vi "LabVIEWArduino1SpreadSheet.vi"() -> ()   [LabVIEW 2020]
uses:
  <vilib>/Instr/_visa.llb/VISA Configure Serial Port (Instr).vi
panel:
  out "FOUND STRING":i32
  out "Element 2":dbl[](array[numeric]) caption="Temperature Array"
  out "Second Element 2":dbl[](graph)
  in  "write buffer":string
  out "GO DOWN ECHO 2":string
  out "GO UP ECHO":string
  in  "GO UP":bool
  in  "GO DOWN":bool
  out "MAX SPEED ECHO":string
  out "SLOW SPEED ECHO":string
  in  "MAX SPEED":bool
  in  "SLOWEST SPEED":bool
  out "First Element":dbl[](graph)
  in  "VISA resource name":refnum<visa-resource-name>="COM3"
  in  "data bits (8)":u16=8 min=5 max=8 step=1
  in  "stop bits (10: 1 bit)":u16(ring)=10 items=["1.0"=10, "1.5"=15, "2.0"=20]
  in  "flow control (0:none)":u16(ring) items=["None", "XON/XOFF", "RTS/CTS", "XON/XOFF & RTS/CTS", "DTR/DSR", "XON/XOFF & DTR/DSR"]
  in  "parity (0:none)":enum16{"None", "Odd", "Even", "Mark", "Space"}(ring)
  out "Element 1":dbl[](array[numeric]) caption="Temperature Array"
  out "concatenated string":string
  in  "stop":bool
  in  "LabVIEW Stop":bool
  out "LabVIEW Echo":string
  out "Emergency Stop Echo":string
  in  "Emergency Stop!":bool
  out "DECELLERATE ECHO":string
  in  "Decellerate":bool
  in  "Motor Control Duino":refnum<visa-resource-name>
  in  "Accelerate":bool
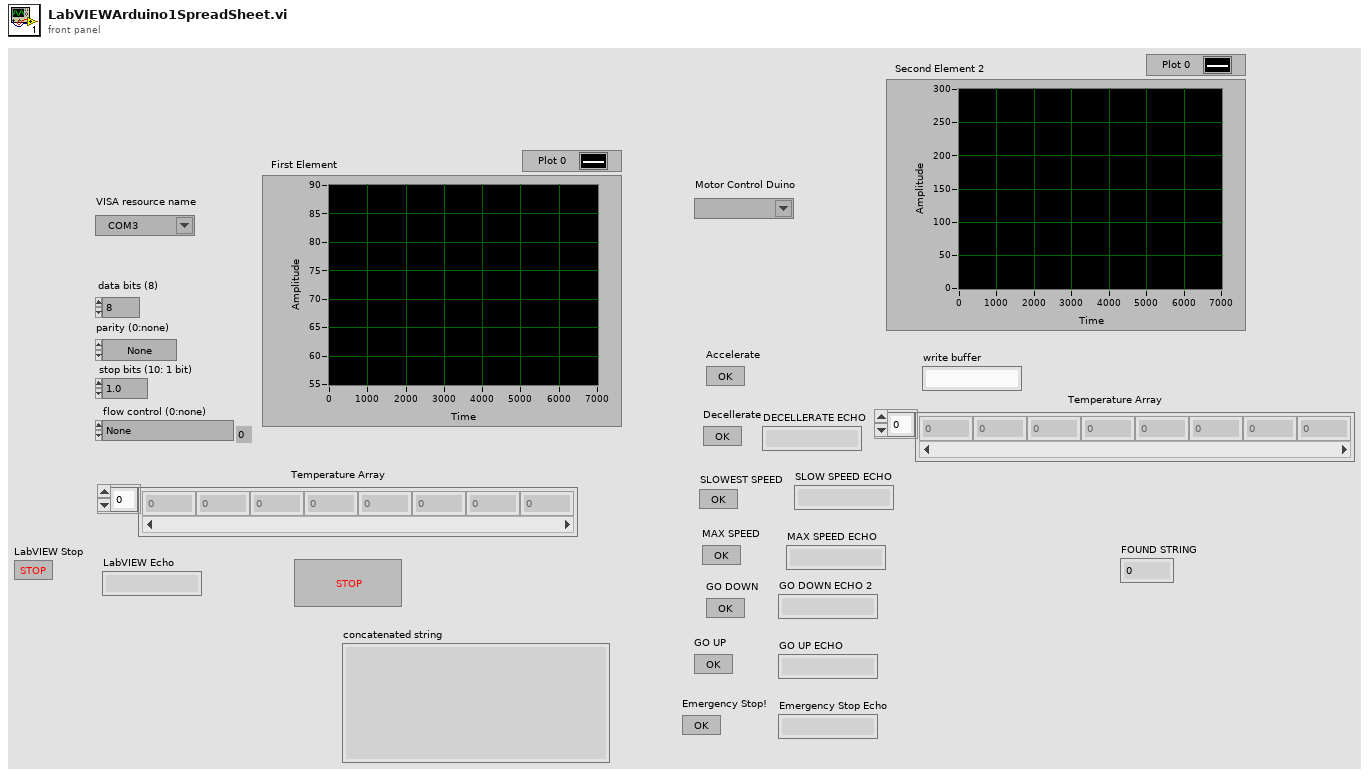
[diagram p1: front panel]
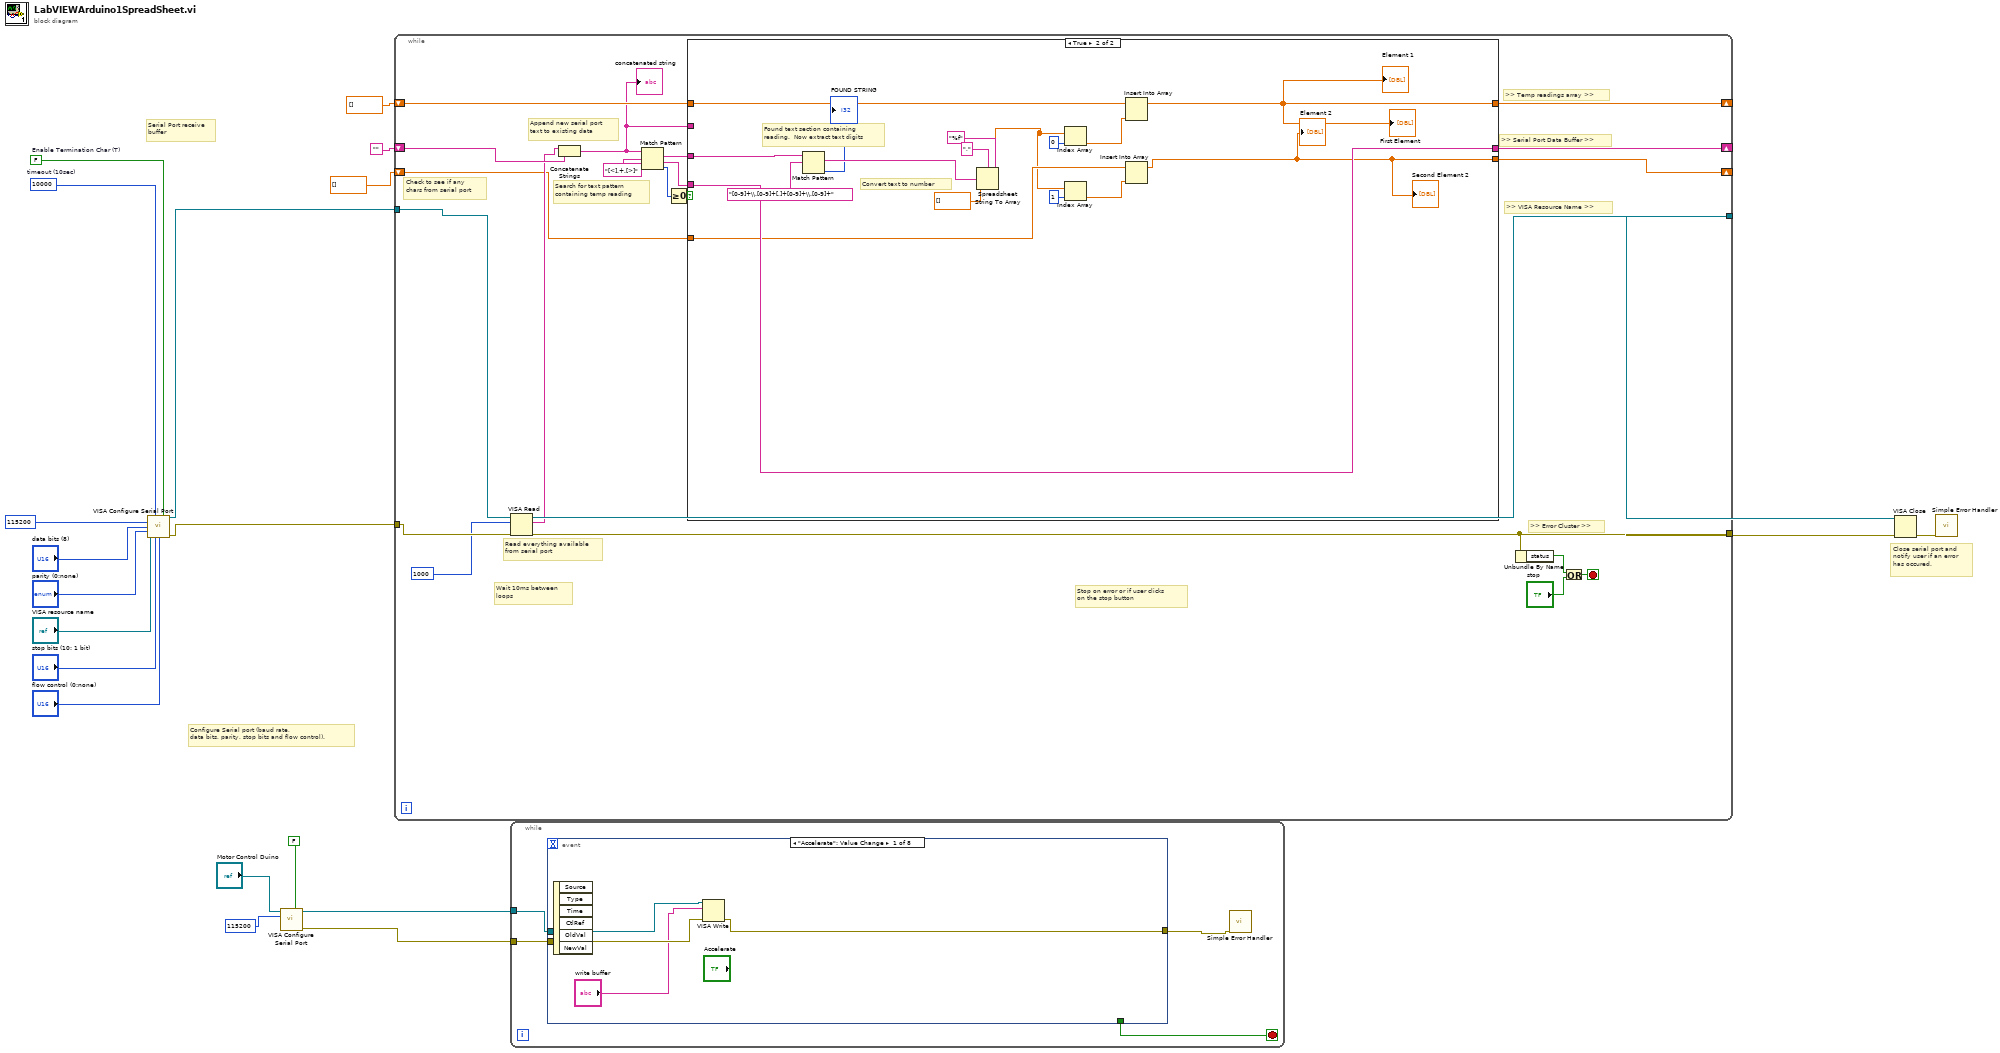
[diagram p0: block diagram]
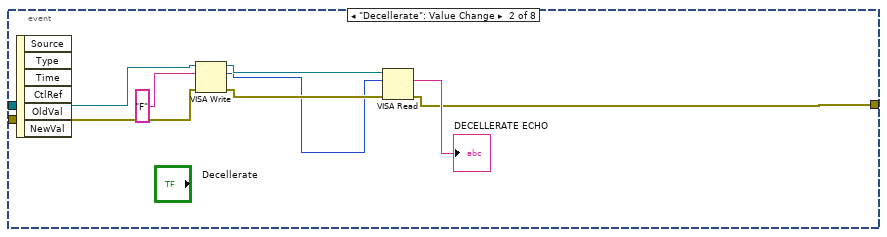
[diagram p3: hidden frame]
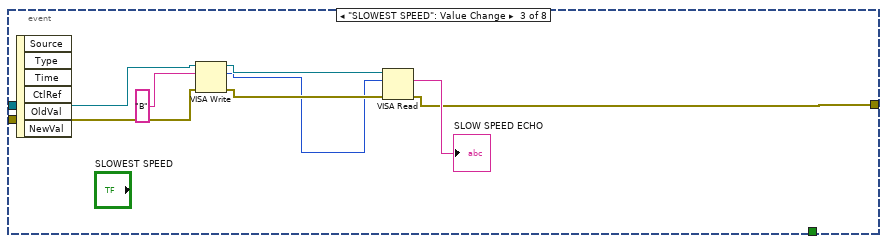
[diagram p4: hidden frame]
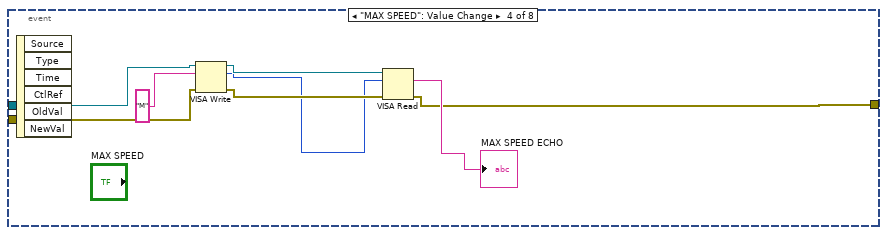
[diagram p5: hidden frame]
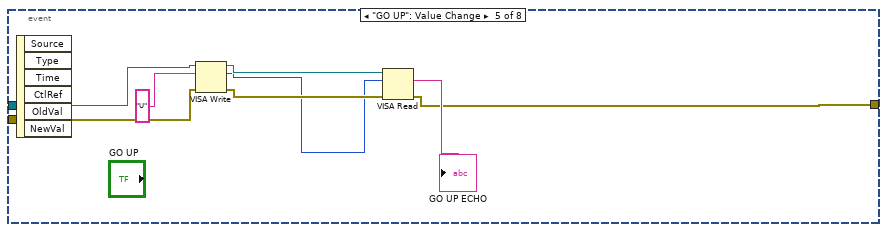
[diagram p6: hidden frame]
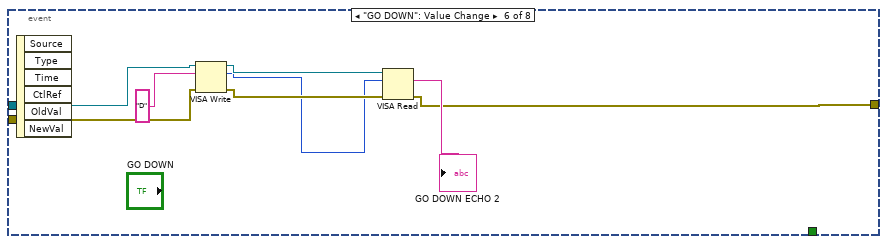
[diagram p7: hidden frame]
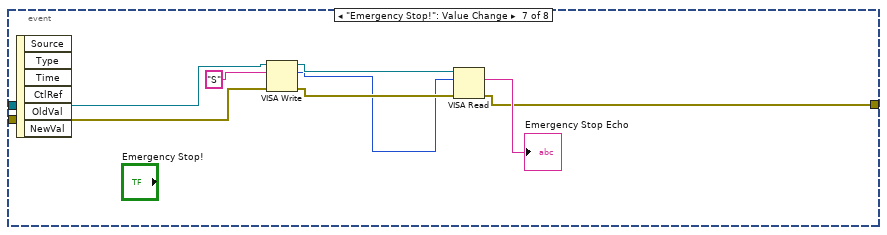
[diagram p8: hidden frame]
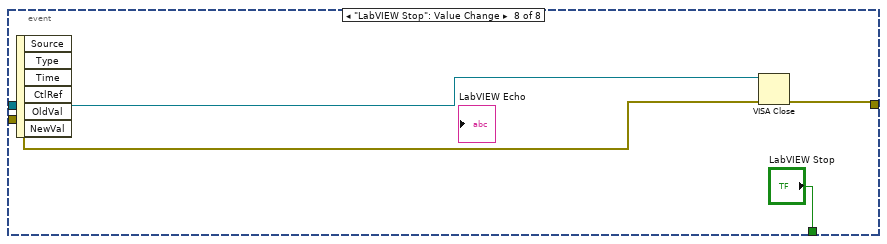
[diagram p9: hidden frame]
diagram:
  w13 = FALSE  # Enable Termination Char (T)
  w14 = u32 10000  # timeout (10sec)
  # "Close serial port and\nnotify user if an error\nhas occured."
  # "Serial Port receive\nbuffer"
  # "Configure Serial port (baud rate,\ndata bits, parity, stop bits and flow control)."
  n1 = call-poly "VISA Configure Serial Port"("VISA resource name"="VISA resource name", "timeout (10sec)"=w14, "Enable Termination\nChar (T)"=w13, "baud rate (9600)"=u32 115200, "data bits (8)"="data bits (8)", "parity (0:none)"="parity (0:none)", "stop bits (10: 1 bit)"="stop bits (10: 1 bit)", "flow control (0:none)"="flow control (0:none)") -> ("VISA resource name out"=w4:refnum<visa-resource-name>, "error out"=w3:errorcluster)  [unwired: 6 in]
  n2 = call-poly "VISA Configure Serial Port"("VISA resource name"="Motor Control Duino", "Enable Termination\nChar (T)"=FALSE ("Enable Termination\nChar (T)"), "baud rate (9600)"=u32 115200) -> ("VISA resource name out"=w21:refnum<visa-resource-name>, "error out"=w20:errorcluster)  [unwired: 11 in]
  n3 = while {
    tunnel: [w40] -> w17
    tunnel: [w42] -> w16
    shift-right: [w34] -> _
    shift-left: "" -> [w41]
    shift-right: [w36] -> _
    shift-left: dbl[] [] -> [w35]
    tunnel: w4 -> [w33]
    tunnel: w3 -> [w32]
    shift-right: [w23] -> _
    shift-left: dbl[] [] -> [w22]
    stop <- w39 stop-if-true
    # "Search for text pattern\ncontaining temp reading"
    # "Append new serial port\ntext to existing data"
    # "Read everything available\nfrom serial port"
    # "Wait 10ms between \nloops"
    # "Stop on error or if user clicks \non the stop button"
    # ">> Error Cluster >>"
    # ">> VISA Resource Name >>"
    # ">> Temp readings array >>"
    # ">> Serial Port Data Buffer >>"
    # "Check to see if any\nchars from serial port"
    n4 = VISA Read(VISA resource name=w33, byte count=u32 1000, error in (no error)=w32) -> (VISA resource name out=w42:refnum<visa-resource-name>, read buffer=w25:string, error out=w40:errorcluster)  [unwired: 1 out]
    n5 = Concatenate Strings(w25, w41) -> (w26:string)
    "concatenated string" <- w26
    n6 = Match Pattern(string=w26, regular expression="[<].+.[>]") -> (match substring=w28:string, after substring=w27:string, offset past match=w30:i32)  [unwired: 1 in, 1 out]
    n7 = Greater Or Equal To 0?(x=w30) -> (x >= 0?=w29:bool)
    n8 = case shown="True" w29 {
      tunnel: w28 -> [_ w61]
      tunnel: w27 -> [_ w62]
      tunnel: w26 -> [w45 _]
      tunnel: [w45 w62] -> w34
      tunnel: [w44 w58] -> w36
      tunnel: w35 -> [w44 w60]
      tunnel: [w43 w49] -> w23
      tunnel: w22 -> [w43 w50]
      frame False {
        # "Did not find text pattern in the buffer.  Try again in the next loop after new data \nhas been received."
      }
      frame True {
        # "Convert text to number"
        # "Found text section containing \nreading.  Now extract text digits"
        n9 = Match Pattern(string=w61, regular expression="[0-9]+\\.[0-9]+[,]+[0-9]+\\.[0-9]+") -> (match substring=w53:string, offset past match=→"FOUND STRING":i32)  [unwired: 1 in, 2 out]
        n10 = Spreadsheet String To Array(delimiter (Tab)=",", format string="%f", spreadsheet string=w53, array type (2D Dbl)=dbl[] []) -> (array=w46:dbl[])
        n11 = Index Array(array=w46, index=0 ("index (row)")) -> (element=w52:dbl)
        n12 = Index Array(array=w46, index=1 ("index (row)")) -> (element=w51:dbl)
        n13 = Insert Into Array(array=w50, new element=w51) -> (w49:dbl[])  [unwired: 1 in]
        "Second Element 2" <- w49
        "Element 2" <- w49
        n14 = Insert Into Array(array=w60, new element=w52) -> (w58:dbl[])  [unwired: 1 in]
        "Element 1" <- w58
        "First Element" <- w58
      }
    }
    n15 = Unbundle By Name(w40) -> ("status"=w38:bool)
    n16 = Or(x=w38, y="stop") -> (x .or. y?=w39:bool)
  }
  n17 = while {
    tunnel: w21 -> [w66]
    tunnel: w20 -> [w65]
    stop <- w63 stop-if-true
    n18 = event shown="[0] \"Accelerate\": Value Change" {
      selector: _ -> [_ _ _ _ _ _ _ _]
      dyn-events: _ -> [_ _ _ _ _ _ _ _]
      timeout: _ -> [_ _ _ _ _ _ _ _]
      tunnel: [w70 w71 w79 w87 w95 w103 w111 w122] -> w64
      tunnel: w66 -> [w69 w73 w81 w89 w97 w105 w113 w121]
      tunnel: w65 -> [w68 w72 w80 w88 w96 w104 w112 w120]
      tunnel: [_ _ _ _ _ _ _ "LabVIEW Stop"] -> w63
      event "Accelerate": Value Change {
        n19 = event-data() -> ()  [unwired: 1 in, 6 out]
        n20 = VISA Write(VISA resource name=w69, write buffer="write buffer", error in (no error)=w68) -> (error out=w70:errorcluster)  [unwired: 2 out]
      }
      event "Decellerate": Value Change {
        n21 = event-data() -> ()  [unwired: 1 in, 6 out]
        n22 = VISA Write(VISA resource name=w73, write buffer="F", error in (no error)=w72) -> (VISA resource name out=w77:refnum<visa-resource-name>, return count=w75:u32, error out=w76:errorcluster)
        n23 = VISA Read(VISA resource name=w77, byte count=w75, error in (no error)=w76) -> (read buffer=→"DECELLERATE ECHO":string, error out=w71:errorcluster)  [unwired: 2 out]
      }
      event "SLOWEST SPEED": Value Change {
        n24 = event-data() -> ()  [unwired: 1 in, 6 out]
        n25 = VISA Write(VISA resource name=w81, write buffer="B", error in (no error)=w80) -> (VISA resource name out=w85:refnum<visa-resource-name>, return count=w83:u32, error out=w84:errorcluster)
        n26 = VISA Read(VISA resource name=w85, byte count=w83, error in (no error)=w84) -> (read buffer=→"SLOW SPEED ECHO":string, error out=w79:errorcluster)  [unwired: 2 out]
      }
      event "MAX SPEED": Value Change {
        n27 = event-data() -> ()  [unwired: 1 in, 6 out]
        n28 = VISA Write(VISA resource name=w89, write buffer="M", error in (no error)=w88) -> (VISA resource name out=w93:refnum<visa-resource-name>, return count=w91:u32, error out=w92:errorcluster)
        n29 = VISA Read(VISA resource name=w93, byte count=w91, error in (no error)=w92) -> (read buffer=→"MAX SPEED ECHO":string, error out=w87:errorcluster)  [unwired: 2 out]
      }
      event "GO UP": Value Change {
        n30 = event-data() -> ()  [unwired: 1 in, 6 out]
        n31 = VISA Write(VISA resource name=w97, write buffer="U", error in (no error)=w96) -> (VISA resource name out=w101:refnum<visa-resource-name>, return count=w99:u32, error out=w100:errorcluster)
        n32 = VISA Read(VISA resource name=w101, byte count=w99, error in (no error)=w100) -> (read buffer=→"GO UP ECHO":string, error out=w95:errorcluster)  [unwired: 2 out]
      }
      event "GO DOWN": Value Change {
        n33 = event-data() -> ()  [unwired: 1 in, 6 out]
        n34 = VISA Write(VISA resource name=w105, write buffer="D", error in (no error)=w104) -> (VISA resource name out=w109:refnum<visa-resource-name>, return count=w107:u32, error out=w108:errorcluster)
        n35 = VISA Read(VISA resource name=w109, byte count=w107, error in (no error)=w108) -> (read buffer=→"GO DOWN ECHO 2":string, error out=w103:errorcluster)  [unwired: 2 out]
      }
      event "Emergency Stop!": Value Change {
        n36 = event-data() -> ()  [unwired: 1 in, 6 out]
        n37 = VISA Write(VISA resource name=w113, write buffer="S", error in (no error)=w112) -> (VISA resource name out=w117:refnum<visa-resource-name>, return count=w115:u32, error out=w116:errorcluster)
        n38 = VISA Read(VISA resource name=w117, byte count=w115, error in (no error)=w116) -> (read buffer=→"Emergency Stop Echo":string, error out=w111:errorcluster)  [unwired: 2 out]
      }
      event "LabVIEW Stop": Value Change {
        n39 = event-data() -> ()  [unwired: 1 in, 6 out]
        n40 = VISA Close(VISA resource name=w121, error in (no error)=w120) -> (error out=w122:errorcluster)
      }
    }
    n41 = call <vilib>:"Simple Error Handler.vi"("error in (no error)"=w64) -> ()  [unwired: 4 in, 5 out]
  }
  n42 = VISA Close(VISA resource name=w16, error in (no error)=w17) -> (error out=w15:errorcluster)
  n43 = call <vilib>:"Simple Error Handler.vi"("error in (no error)"=w15) -> ()  [unwired: 4 in, 5 out]
